vi "Bairstow_Relative Error.vi"(8 "threshold":dbl, 9 "dx/x in":dbl, 10 "x":dbl, 11 "dx":dbl) -> (2 "less eps":bool, 3 "dx/x out":dbl)   [LabVIEW 2017, in "NI_AALPro.lvlib"]
uses:
  NI_AALPro.lvlib
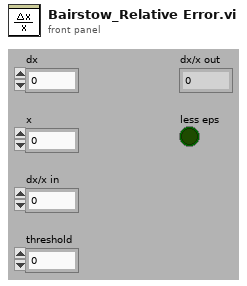
[diagram p1: front panel]
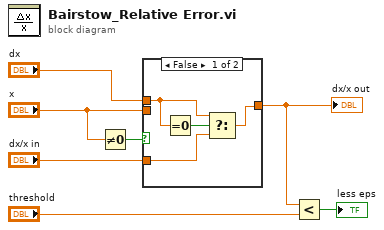
[diagram p0: block diagram]
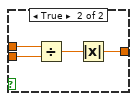
[diagram p2: hidden frame]
diagram:
  n1 = Not Equal To 0?(x="x") -> (x != 0?=w6:bool)
  n2 = case shown="False" w6 {
    tunnel: "dx" -> [w9 w15]
    tunnel: "x" -> [_ w14]
    tunnel: "dx/x in" -> [w10 _]
    tunnel: [w8 w12] -> w3
    frame False {
      n3 = Equal To 0?(x=w9) -> (x = 0?=w11:bool)
      n4 = Select(t=w9, s=w11, f=w10) -> (s? t:f=w8:dbl)
    }
    frame True {
      n5 = Divide(x=w15, y=w14) -> (x/y=w13:dbl)
      n6 = Absolute Value(x=w13) -> (abs(x)=w12:dbl)
    }
  }
  "dx/x out" <- w3
  n7 = Less?(x=w3, y="threshold") -> (x < y?=→"less eps":bool)
